vi "CRYDelete Step Data.vi"(11 "Step No":i32[](array[numeric])) -> ()   [LabVIEW 2013]
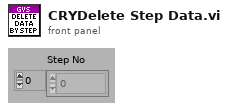
[diagram p1: front panel]
types:
  T1 = typedef "CRYData Cluster.ctl" = cluster{"Name":string, "Curve":cluster{"x":dbl, "y":dbl, "z":dbl}[], "X data":u16, "Y data":u16, "Z data":u16, "X axis":u16, "Y axis":u16, "Z axis":u16, "X unit":string, "Y unit":string, "Z unit":string, "X dB ref":dbl, "Y dB ref":dbl, "Z dB ref":dbl, "single val":bool, "protected":bool, "display X":bool, "display Y":bool, "display Z":bool, "Test Info":string, "Step No.":i32, "Plot Settings":cluster{"Color":u32, "Interpolation":u8, "Point Style":u8, "Line Style":u8, "Point Color":u32, "Line Width":u8, "Bar Plot Style":u8, "Fill To":i16}, "AutoProtect":bool}
  T2 = typedef "CRYWaveform Cluster.ctl" = cluster{"Waveform":cluster{"X0":dbl, "dX":dbl, "Y":sgl[]}, "X data":u16, "Y data":u16, "Y axis":u16, "X unit":string, "Y unit":string, "Y dB ref":dbl, "display Y":bool, "display X":bool, "Overload?":bool, "Test Info":string, "Step No.":i32, "Name":string, "protected":bool, "Sqc history":string[], "Signal Channel ID":i32, "Plot Settings":cluster{"Color":u32, "Interpolation":u8, "Point Style":u8, "Line Style":u8, "Point Color":u32, "Line Width":u8, "Bar Plot Style":u8, "Fill To":i16}, "AutoProtect":bool}
  T3 = typedef "CRYResult Cluster.ctl" = cluster{"Name":string, "Margin":dbl, "unit":string, "Verdict":bool, "Limit":string, "Max/Min":string, "protected":bool, "Step No.":i32, "Test Info":string, "AutoProtect":bool}
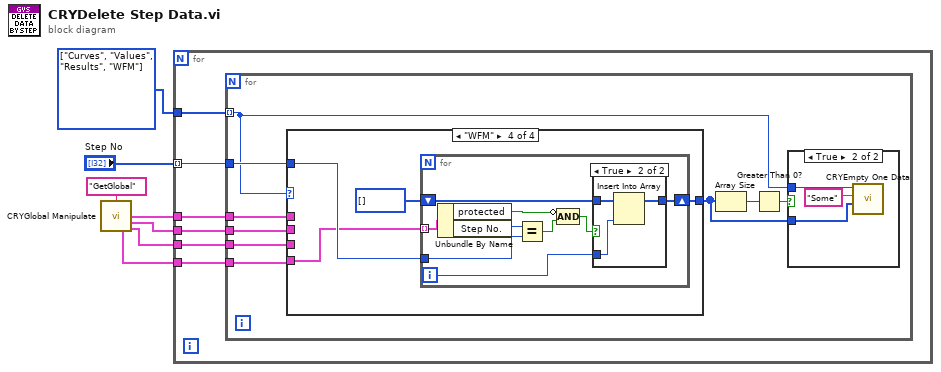
[diagram p0: block diagram]
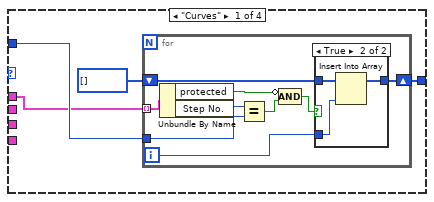
[diagram p3: hidden frame]
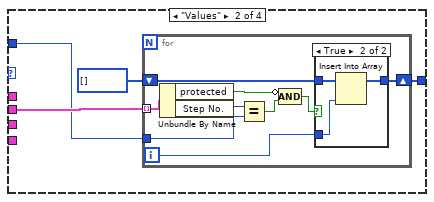
[diagram p5: hidden frame]
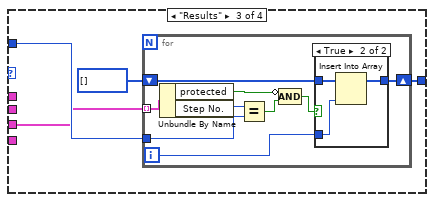
[diagram p7: hidden frame]
diagram:
  w1 = enum16{"Curves", "Values", "Results", "WFM"}[] [enum."Curves", enum."Values", enum."Results", enum."WFM"] items=["Curves", "Values", "Results", "WFM"]
  n1 = call "CRYGlobal Manipulate.vi"("sAction"="GetGlobal") -> ("Curves Out"=w5:T1[], "Values Out"=w4:T1[], "WFM Out"=w2:T2[], "Results Out"=w3:T3[])  [unwired: 8 in, 3 out]
  n2 = for {
    tunnel: "Step No" -> [w13] mode=indexing
    tunnel: w5 -> [w11]
    tunnel: w4 -> [w10]
    tunnel: w3 -> [w9]
    tunnel: w2 -> [w8]
    tunnel: w1 -> [w12]
    n3 = for {
      tunnel: w12 -> [w19] mode=indexing
      tunnel: w13 -> [w22]
      tunnel: w11 -> [w17]
      tunnel: w10 -> [w16]
      tunnel: w9 -> [w15]
      tunnel: w8 -> [w14]
      n4 = case shown="\"WFM\"" w19 {
        tunnel: w16 -> [_ w46 _ _]
        tunnel: w15 -> [_ _ w60 _]
        tunnel: w14 -> [_ _ _ w77]
        tunnel: w22 -> [w29 w45 w63 w80]
        tunnel: [w28 w44 w62 w79] -> w18
        tunnel: w17 -> [w26 _ _ _]
        frame "Curves" {
          n5 = for {
            tunnel: w26 -> [w38] mode=indexing
            tunnel: w29 -> [w36]
            shift-right: [w35] -> w28
            shift-left: i32[] [] -> [w34]
            i -> [w33]
            n6 = Unbundle By Name(w38) -> ("protected"=w32:bool, "Step No."=w37:i32)
            n7 = Equal?(x=w37, y=w36) -> (x = y?=w31:bool)
            n8 = Compound Arithmetic op=AND(invert w32, w31) -> (w30:bool)
            n9 = case shown="True" w30 {
              tunnel: [w39 w42] -> w35
              tunnel: w34 -> [w39 w41]
              tunnel: w33 -> [_ w40]
              frame False {
              }
              frame True {
                n10 = Insert Into Array(array=w41, new element=w40) -> (w42:i32[])  [unwired: 1 in]
              }
            }
          }
        }
        frame "Values" {
          n11 = for {
            tunnel: w46 -> [w55] mode=indexing
            tunnel: w45 -> [w53]
            shift-right: [w52] -> w44
            shift-left: i32[] [] -> [w51]
            i -> [w50]
            n12 = Unbundle By Name(w55) -> ("protected"=w49:bool, "Step No."=w54:i32)
            n13 = Equal?(x=w54, y=w53) -> (x = y?=w48:bool)
            n14 = Compound Arithmetic op=AND(invert w49, w48) -> (w47:bool)
            n15 = case shown="True" w47 {
              tunnel: [w56 w59] -> w52
              tunnel: w51 -> [w56 w58]
              tunnel: w50 -> [_ w57]
              frame False {
              }
              frame True {
                n16 = Insert Into Array(array=w58, new element=w57) -> (w59:i32[])  [unwired: 1 in]
              }
            }
          }
        }
        frame "Results" {
          n17 = for {
            tunnel: w60 -> [w72] mode=indexing
            tunnel: w63 -> [w70]
            shift-right: [w69] -> w62
            shift-left: i32[] [] -> [w68]
            i -> [w67]
            n18 = Unbundle By Name(w72) -> ("protected"=w66:bool, "Step No."=w71:i32)
            n19 = Equal?(x=w71, y=w70) -> (x = y?=w65:bool)
            n20 = Compound Arithmetic op=AND(invert w66, w65) -> (w64:bool)
            n21 = case shown="True" w64 {
              tunnel: [w73 w76] -> w69
              tunnel: w68 -> [w73 w75]
              tunnel: w67 -> [_ w74]
              frame False {
              }
              frame True {
                n22 = Insert Into Array(array=w75, new element=w74) -> (w76:i32[])  [unwired: 1 in]
              }
            }
          }
        }
        frame "WFM" {
          n23 = for {
            tunnel: w77 -> [w89] mode=indexing
            tunnel: w80 -> [w87]
            shift-right: [w86] -> w79
            shift-left: i32[] [] -> [w85]
            i -> [w84]
            n24 = Unbundle By Name(w89) -> ("protected"=w83:bool, "Step No."=w88:i32)
            n25 = Equal?(x=w88, y=w87) -> (x = y?=w82:bool)
            n26 = Compound Arithmetic op=AND(invert w83, w82) -> (w81:bool)
            n27 = case shown="True" w81 {
              tunnel: [w90 w93] -> w86
              tunnel: w85 -> [w90 w92]
              tunnel: w84 -> [_ w91]
              frame False {
              }
              frame True {
                n28 = Insert Into Array(array=w92, new element=w91) -> (w93:i32[])  [unwired: 1 in]
              }
            }
          }
        }
      }
      n29 = Array Size(array=w18) -> (size(s)=w21:i32)
      n30 = Greater Than 0?(x=w21) -> (x > 0?=w20:bool)
      n31 = case shown="True" w20 {
        tunnel: w19 -> [_ w25]
        tunnel: w18 -> [_ w23]
        frame False {
        }
        frame True {
          n32 = call "CRYEmpty One Data.vi"("Index"=w23, "sOption"="Some", "Type"=w25) -> ()  [unwired: 9 in]
        }
      }
    }
  }
